vi "Spin Image.vi"(8 "error in (no error)":errorcluster, 10 "data":sgl[](array[numeric]), 11 "image data IN":T1) -> (0 "error out":errorcluster, 2 "image":picture, 3 "image data OUT":T1)   [LabVIEW 2017, in "process_Angle.lvlib"]
uses:
  process_Angle.lvlib
  image_vi/image.lvlib
  <vilib>/picture/picture.llb/imagedata.ctl
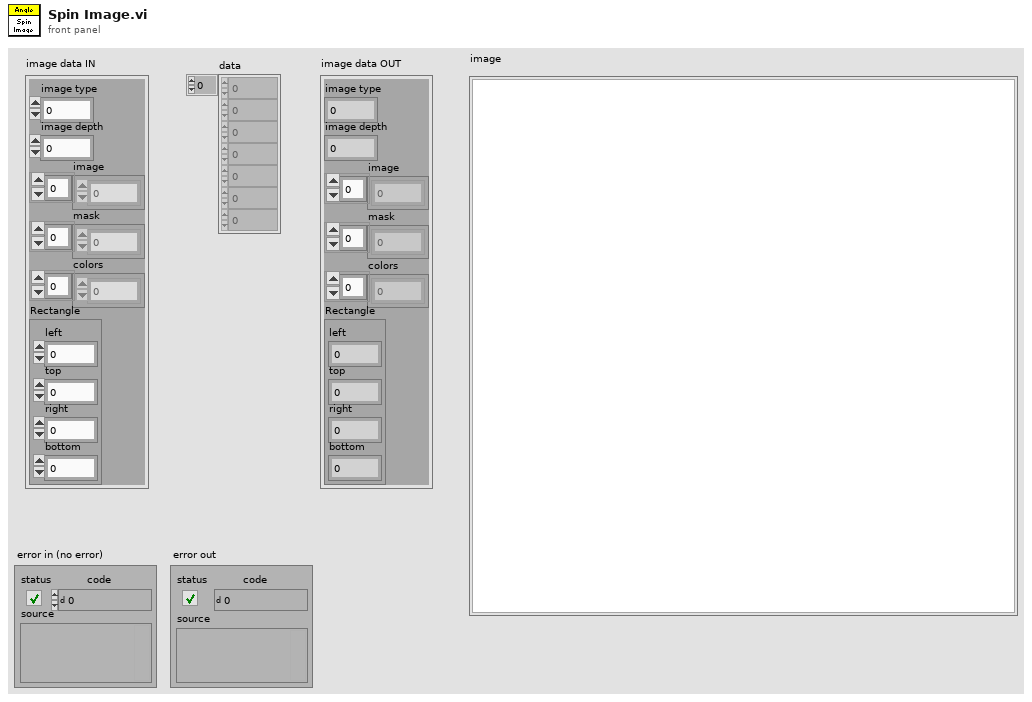
[diagram p1: front panel]
types:
  T1 = typedef "imagedata.ctl" = cluster{"image type":i32, "image depth":i32, "image":u8[], "mask":u8[], "colors":u32[], "Rectangle":cluster{"left":i16, "top":i16, "right":i16, "bottom":i16}}
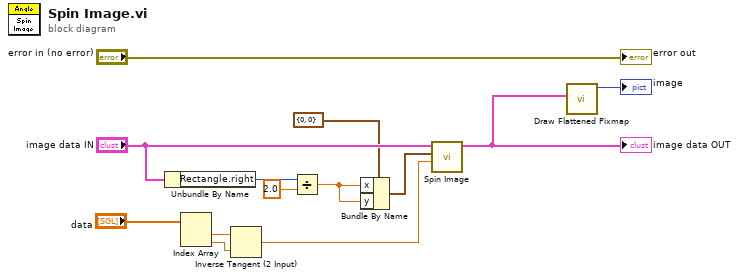
[diagram p0: block diagram]
diagram:
  n1 = Unbundle By Name("image data IN") -> ("Rectangle.right"=w5:i16)
  n2 = Index Array(array="data") -> (element #1=w12:sgl, element #2=w11:sgl)  [unwired: 2 in]
  n3 = Inverse Tangent (2 Input)(1:w11, 2:w12) -> (0:w7:sgl)
  n4 = Divide(x=w5, y=2.0) -> (x/y=w2:dbl)
  n5 = Bundle By Name(cluster=cluster{"x":i16, "y":i16} {"x"=0, "y"=0} ("RotationPoint"), "x"=w2, "y"=w2) -> (w1:cluster{"x":i16, "y":i16})
  n6 = call "Spin Image.vi"("Angle [rad]"=w7, "RotationPoint"=w1, "Image In"="image data IN") -> ("Image Out"=w9:T1)  [unwired: 8 in]
  "image data OUT" <- w9
  n7 = call <vilib>:"Draw Flattened Pixmap.vi"("image data"=w9) -> ("new picture"=→"image":picture)  [unwired: 8 in]
  "error out" <- "error in (no error)"
